vi "HRV_EEG_version4.vi"() -> ()   [LabVIEW 2014]
uses:
  <vilib>/Utility/file.llb/Read From Spreadsheet File (I64).vi
  <vilib>/Utility/file.llb/Write To Spreadsheet File (DBL).vi
panel:
  out "size(s) 3":i32[](array[numeric])
  out "size(s) 2":i32
  out "size(s)":i32[](array[numeric])
  out "Trial_Number":i64
  out "created path":path
  out "error out":errorcluster
  in  "피험자_이름":string="김다영"
  out "PPI+ERP":dbl[][](graph)
  out "HF+ERP":dbl[][](graph)
  out "LF+ERP":dbl[][](graph)
  out "VLF+ERP":dbl[][](graph)
  out "PPI":dbl[][](graph)
  in  "PPI":path=path "C:/Users/Jaehong/Desktop/Classifiers/HRV_EEG/NewData/김다영_PPI.txt"
  in  "HF":path=path "C:/Users/Jaehong/Desktop/Classifiers/HRV_EEG/NewData/김다영_HF.txt"
  in  "LF":path=path "C:/Users/Jaehong/Desktop/Classifiers/HRV_EEG/NewData/김다영_LF.txt"
  in  "VLF":path=path "C:/Users/Jaehong/Desktop/Classifiers/HRV_EEG/NewData/김다영_VLF.txt"
  out "HF":dbl[][](graph)
  out "LF":dbl[][](graph)
  out "VLF":dbl[][](graph)
  out "Target_icon":i64
  in  "Target_Total":path=path "C:/Users/Jaehong/Desktop/Classifiers/data/통합LDAs/김다영/target_order.txt"
  out "ERP_Graph":dbl[][](graph)
  in  "ERP_Total":path=path "C:/Users/Jaehong/Desktop/Classifiers/HRV_EEG/ERP_total/김다영/ERP_total.txt"
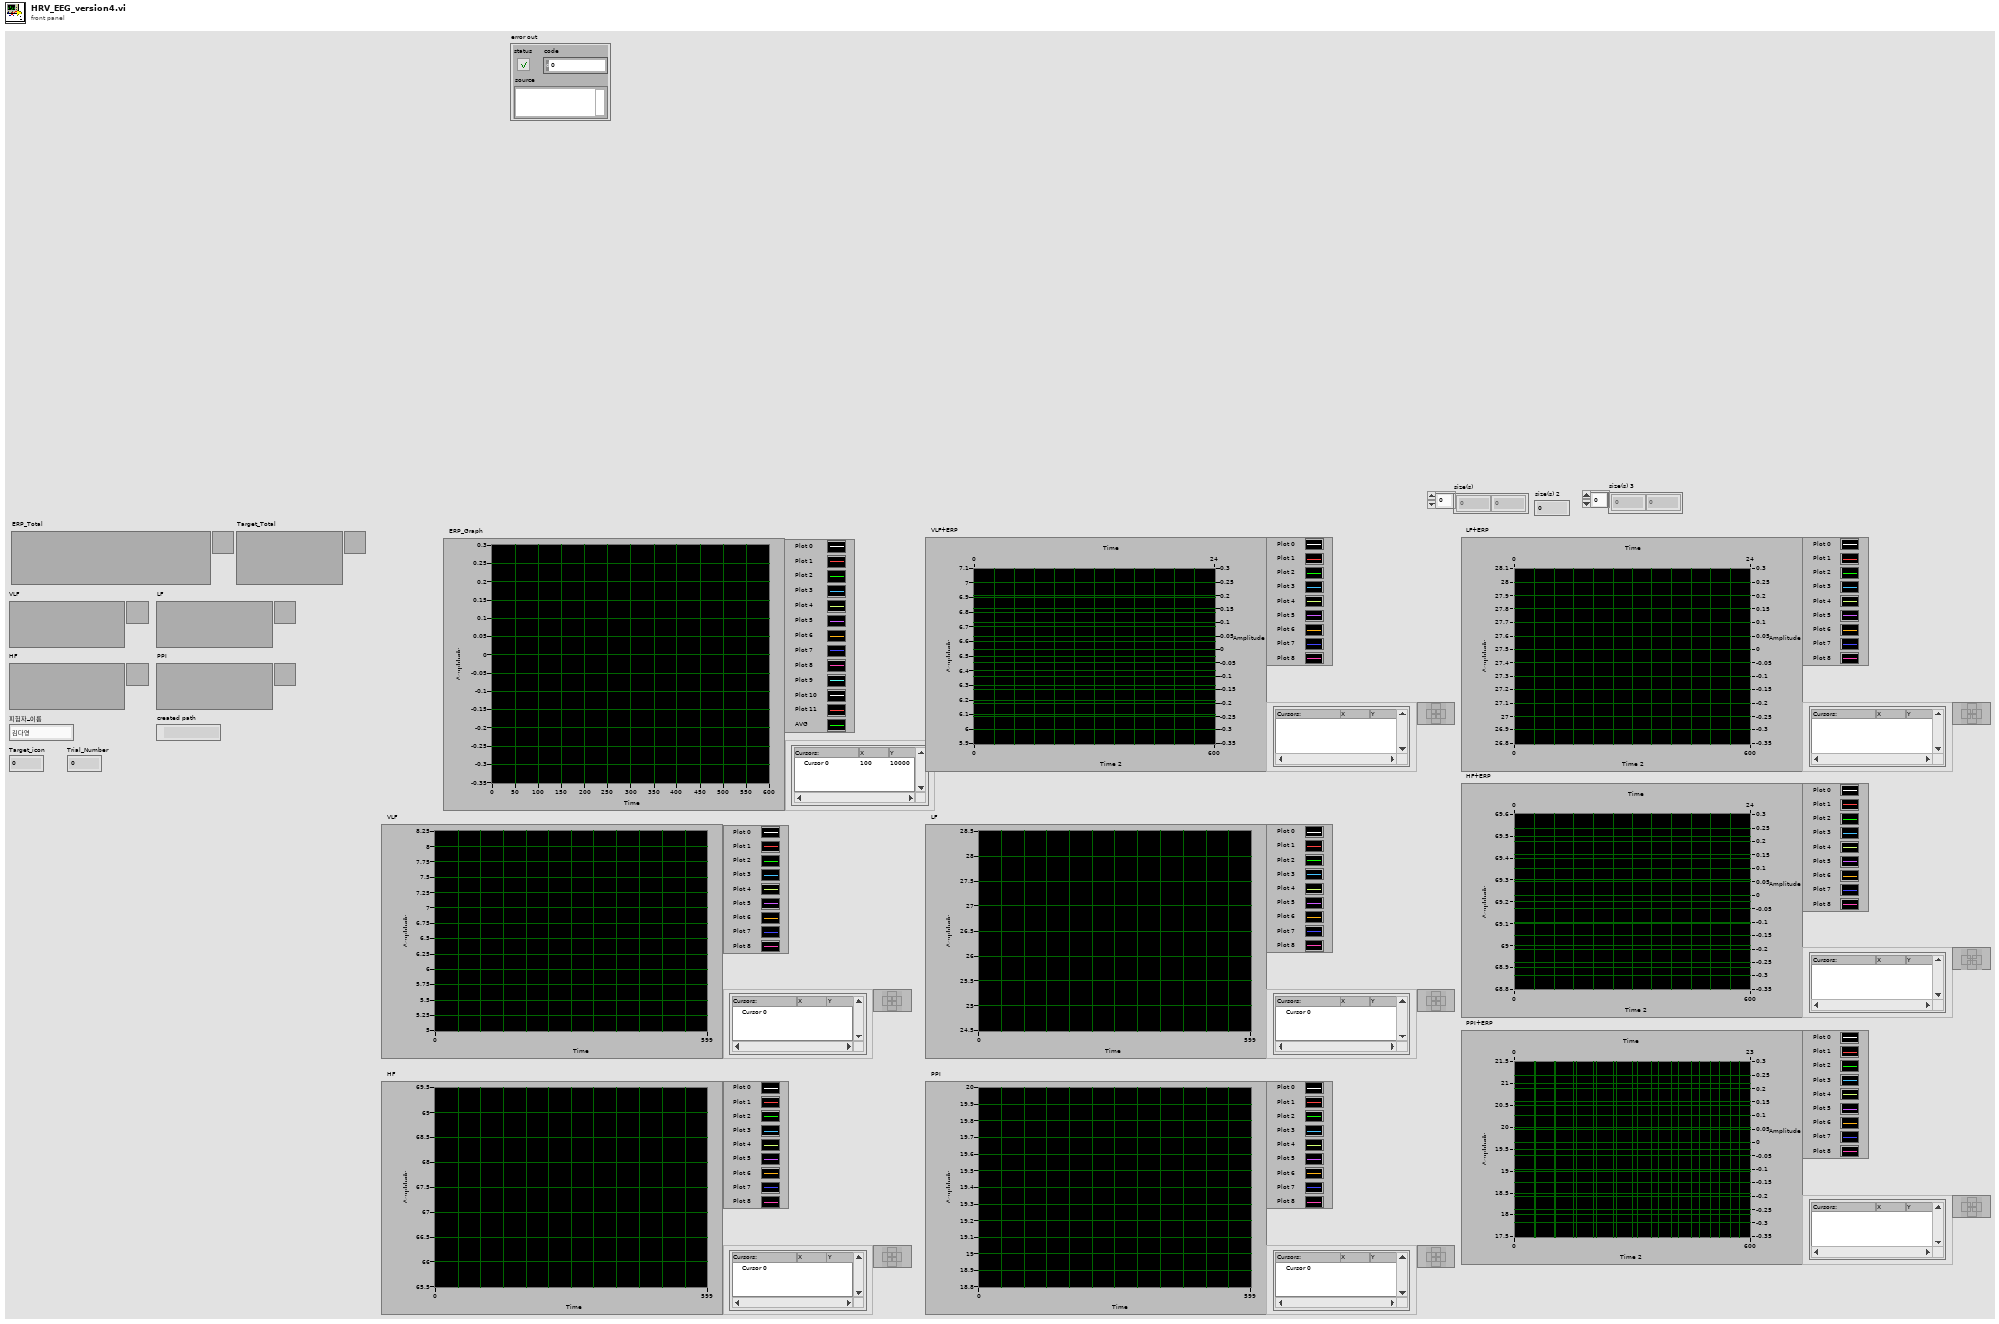
[diagram p1: front panel]
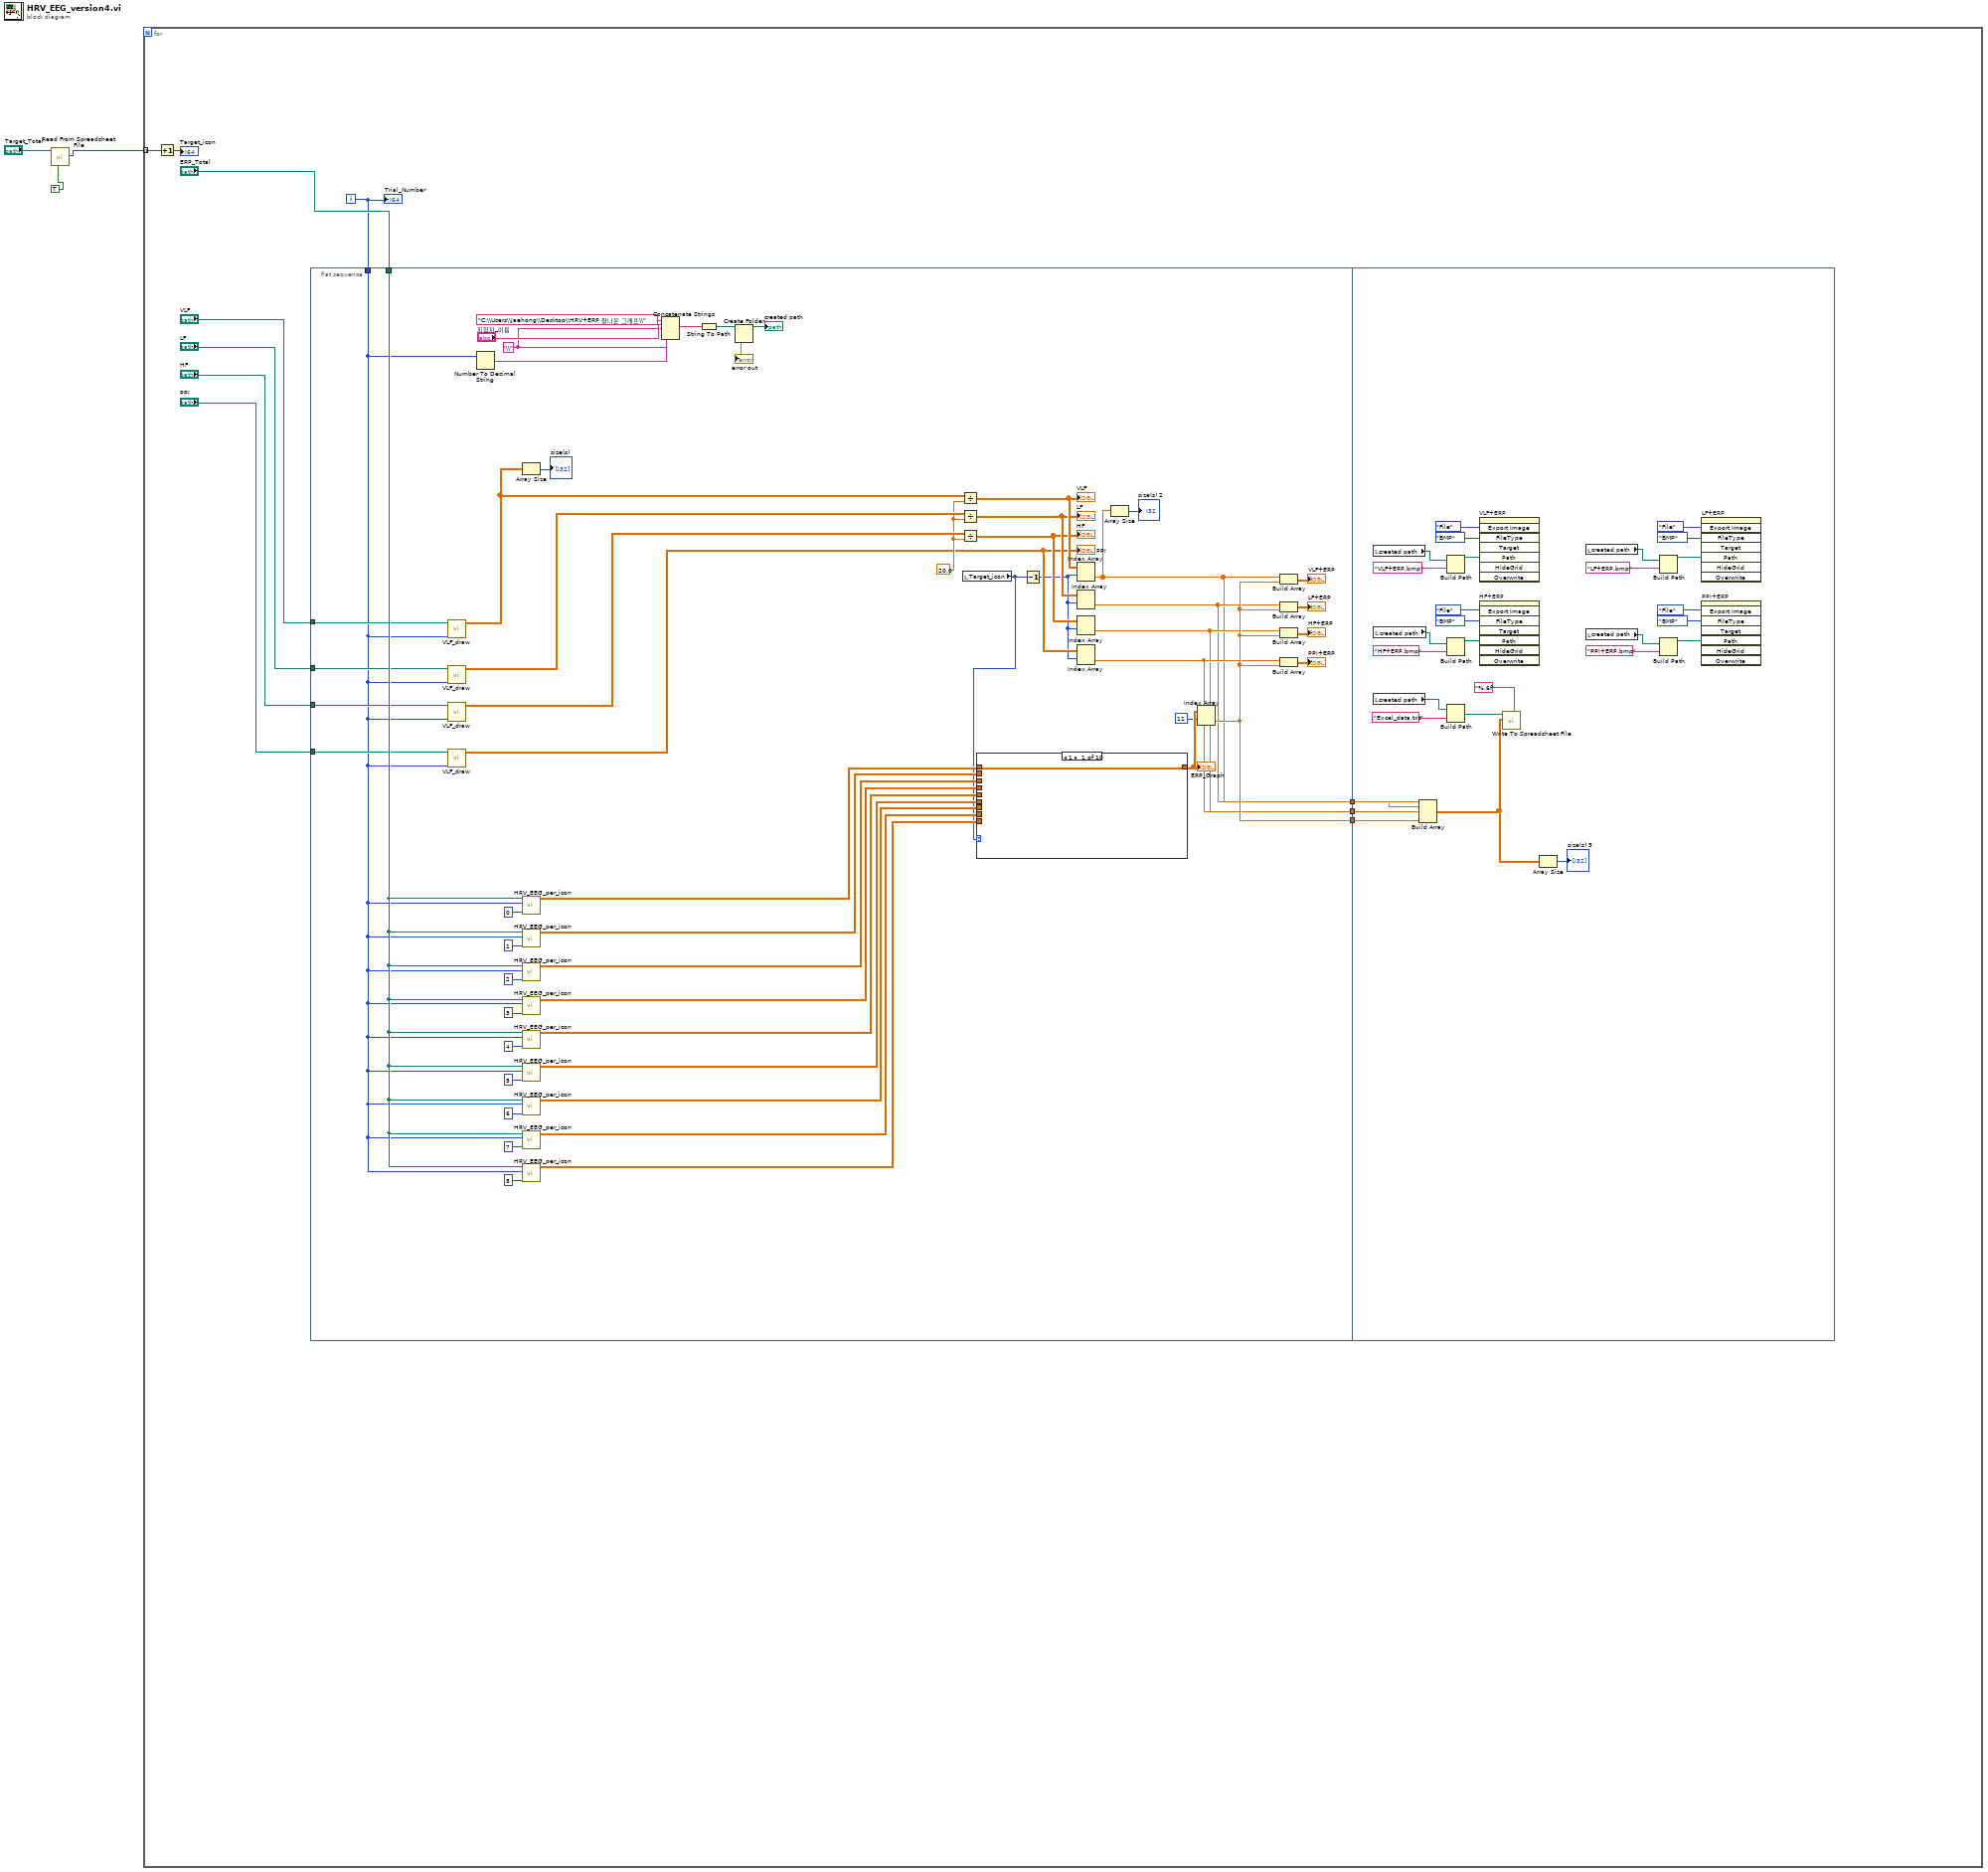
[diagram p0: block diagram]
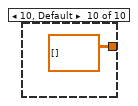
[diagram p10: hidden frame]
diagram:
  n1 = call-poly <vilib>:"Read From Spreadsheet File.vi"("transpose (no:F)"=TRUE, "file path (dialog if empty)"="Target_Total") -> ("first row"=w2:i64[])  [unwired: 5 in, 4 out]
  n2 = for {
    tunnel: w2 -> [w4] mode=indexing
    i -> [w5]
    n3 = Increment(x=w4) -> (x+1=→"Target_icon":i64)
    n4 = flat-sequence {
      tunnel: w5 -> [w17]
      tunnel: "ERP_Total" -> [w65]
      tunnel: "VLF" -> [w62]
      tunnel: "LF" -> [w61]
      tunnel: "HF" -> [w60]
      tunnel: "PPI" -> [w59]
      tunnel: [w18] -> w10
      tunnel: [w19] -> w9
      tunnel: [w20] -> w8
      tunnel: [w21] -> w7
      tunnel: [w27] -> w6
      tunnel: w10 -> [w92]
      tunnel: w9 -> [w91]
      tunnel: w8 -> [w90]
      tunnel: w7 -> [w89]
      tunnel: w6 -> [w88]
      frame #0 {
        w38 = "\\"
        w56 = 20.0
        n5 = call "VLF_draw.vi"("Trial_Number"=w17, "HRV(VLF, LF, HF, PPI)"=w62) -> ("Icon1"=w24:dbl[][])  [unwired: 9 in]
        n6 = call "VLF_draw.vi"("Trial_Number"=w17, "HRV(VLF, LF, HF, PPI)"=w61) -> ("Icon1"=w58:dbl[][])  [unwired: 9 in]
        n7 = call "VLF_draw.vi"("Trial_Number"=w17, "HRV(VLF, LF, HF, PPI)"=w60) -> ("Icon1"=w57:dbl[][])  [unwired: 9 in]
        n8 = call "VLF_draw.vi"("Trial_Number"=w17, "HRV(VLF, LF, HF, PPI)"=w59) -> ("Icon1"=w49:dbl[][])  [unwired: 9 in]
        "PPI" <- w49
        n9 = Number To Decimal String(number=w17) -> (decimal integer string=w42:string)  [unwired: 1 in]
        n10 = call "HRV_EEG_per_icon.vi"("Icon Number"=0, "Trial_Number"=w17, "ERP_Total"=w65) -> ("Icon1"=w55:dbl[][])  [unwired: 8 in]
        n11 = call "HRV_EEG_per_icon.vi"("Icon Number"=1, "Trial_Number"=w17, "ERP_Total"=w65) -> ("Icon1"=w71:dbl[][])  [unwired: 8 in]
        n12 = call "HRV_EEG_per_icon.vi"("Icon Number"=2, "Trial_Number"=w17, "ERP_Total"=w65) -> ("Icon1"=w70:dbl[][])  [unwired: 8 in]
        n13 = call "HRV_EEG_per_icon.vi"("Icon Number"=3, "Trial_Number"=w17, "ERP_Total"=w65) -> ("Icon1"=w69:dbl[][])  [unwired: 8 in]
        n14 = call "HRV_EEG_per_icon.vi"("Icon Number"=4, "Trial_Number"=w17, "ERP_Total"=w65) -> ("Icon1"=w64:dbl[][])  [unwired: 8 in]
        n15 = call "HRV_EEG_per_icon.vi"("Icon Number"=5, "Trial_Number"=w17, "ERP_Total"=w65) -> ("Icon1"=w68:dbl[][])  [unwired: 8 in]
        n16 = call "HRV_EEG_per_icon.vi"("Icon Number"=6, "Trial_Number"=w17, "ERP_Total"=w65) -> ("Icon1"=w67:dbl[][])  [unwired: 8 in]
        n17 = call "HRV_EEG_per_icon.vi"("Icon Number"=7, "Trial_Number"=w17, "ERP_Total"=w65) -> ("Icon1"=w63:dbl[][])  [unwired: 8 in]
        n18 = call "HRV_EEG_per_icon.vi"("Icon Number"=8, "Trial_Number"=w17, "ERP_Total"=w65) -> ("Icon1"=w66:dbl[][])  [unwired: 8 in]
        n19 = Array Size(array=w24) -> (size(s)=→"size(s)":i32[])
        n20 = Concatenate Strings("C:\\Users\\Jaehong\\Desktop\\HRV+ERP 잘나온 그래프\\", "피험자_이름", w38, w42, w38) -> (w40:string)
        n21 = String To Path(string=w40) -> (path=w39:path)
        n22 = Create Folder(path (use dialog)=w39) -> (created path=→"created path":path, error out=→"error out":errorcluster)  [unwired: 2 in, 1 out]
        n23 = Divide(x=w24, y=w56) -> (x/y=w52:dbl[][])
        "VLF" <- w52
        n24 = Divide(x=w58, y=w56) -> (x/y=w51:dbl[][])
        "LF" <- w51
        n25 = Divide(x=w57, y=w56) -> (x/y=w50:dbl[][])
        "HF" <- w50
        n26 = local read "Target_icon"() -> (w25:i64)
        n27 = case shown="1" w25 {
          tunnel: w55 -> [w72 _ _ _ _ _ _ _ _ _]
          tunnel: w71 -> [_ w73 _ _ _ _ _ _ _ _]
          tunnel: w70 -> [_ _ w74 _ _ _ _ _ _ _]
          tunnel: w69 -> [_ _ _ w75 _ _ _ _ _ _]
          tunnel: w64 -> [_ _ _ _ w76 _ _ _ _ _]
          tunnel: w68 -> [_ _ _ _ _ w77 _ _ _ _]
          tunnel: w67 -> [_ _ _ _ _ _ w78 _ _ _]
          tunnel: w63 -> [_ _ _ _ _ _ _ w79 _ _]
          tunnel: w66 -> [_ _ _ _ _ _ _ _ w80 _]
          tunnel: [w72 w73 w74 w75 w76 w77 w78 w79 w80 dbl[][] [] ("Icon1")] -> w54
          frame 1 {
          }
          frame 2 {
          }
          frame 3 {
          }
          frame 4 {
          }
          frame 5 {
          }
          frame 6 {
          }
          frame 7 {
          }
          frame 8 {
          }
          frame 9 {
          }
          frame 10, Default {
          }
        }
        "ERP_Graph" <- w54
        n28 = Decrement(x=w25) -> (x-1=w26:i64)
        n29 = Index Array(array=w52, index (row)=w26) -> (element=w18:dbl[])  [unwired: 1 in]
        n30 = Index Array(array=w51, index (row)=w26) -> (element=w19:dbl[])  [unwired: 1 in]
        n31 = Index Array(array=w50, index (row)=w26) -> (element=w20:dbl[])  [unwired: 1 in]
        n32 = Index Array(array=w49, index (row)=w26) -> (element=w21:dbl[])  [unwired: 1 in]
        n33 = Array Size(array=w18) -> (size(s)=→"size(s) 2":i32)
        n34 = Index Array(array=w54, index (row)=11) -> (element=w27:dbl[])  [unwired: 1 in]
        n35 = Build Array(w18, w27) -> (→"VLF+ERP":dbl[][])
        n36 = Build Array(w19, w27) -> (→"LF+ERP":dbl[][])
        n37 = Build Array(w20, w27) -> (→"HF+ERP":dbl[][])
        n38 = Build Array(w21, w27) -> (→"PPI+ERP":dbl[][])
      }
      frame #1 {
        n39 = local read "created path"() -> (w100:path)
        n40 = local read "created path"() -> (w87:path)
        n41 = local read "created path"() -> (w99:path)
        n42 = Build Array(w92, w91, w90, w89, w88) -> (w82:dbl[][])
        n43 = Build Path(base path=w100, name or relative path="VLF+ERP.bmp") -> (appended path=w108:path)
        n44 = Build Path(base path=w99, name or relative path="HF+ERP.bmp") -> (appended path=w107:path)
        n45 = Build Path(base path=w87, name or relative path="Excel_data.txt") -> (appended path=w85:path)
        n46 = invoke on="VLF+ERP" class="WFGraph (strict)" method="Export Image"("FileType"=enum32{"BMP", "EPS", "EMF", "PICT"}."BMP" ("File Type"), "Target"=enum32{"File", "Clipboard"}."File", "Path"=w108) -> ()  [unwired: 5 in, 8 out]
        n47 = invoke on="HF+ERP" class="WFGraph (strict)" method="Export Image"("FileType"=enum32{"BMP", "EPS", "EMF", "PICT"}."BMP" ("File Type"), "Target"=enum32{"File", "Clipboard"}."File", "Path"=w107) -> ()  [unwired: 5 in, 8 out]
        n48 = call-poly <vilib>:"Write To Spreadsheet File.vi"("format (%.3f)"="%.6f", "2D data"=w82, "file path (dialog if empty)"=w85) -> ()  [unwired: 5 in, 1 out]
        n49 = Array Size(array=w82) -> (size(s)=→"size(s) 3":i32[])
        n50 = local read "created path"() -> (w97:path)
        n51 = local read "created path"() -> (w98:path)
        n52 = Build Path(base path=w97, name or relative path="LF+ERP.bmp") -> (appended path=w103:path)
        n53 = Build Path(base path=w98, name or relative path="PPI+ERP.bmp") -> (appended path=w101:path)
        n54 = invoke on="LF+ERP" class="WFGraph (strict)" method="Export Image"("FileType"=enum32{"BMP", "EPS", "EMF", "PICT"}."BMP" ("File Type"), "Target"=enum32{"File", "Clipboard"}."File", "Path"=w103) -> ()  [unwired: 5 in, 8 out]
        n55 = invoke on="PPI+ERP" class="WFGraph (strict)" method="Export Image"("FileType"=enum32{"BMP", "EPS", "EMF", "PICT"}."BMP" ("File Type"), "Target"=enum32{"File", "Clipboard"}."File", "Path"=w101) -> ()  [unwired: 5 in, 8 out]
      }
    }
    "Trial_Number" <- w5
  }
